vi "PathSearch.vi"(4 "Look-Ahead Time (s)":dbl=0.25, 6 "Search Window (s)":dbl=2.0, 8 "Robot Y (in)":dbl, 9 "Robot X (in)":dbl, 11 "Path":dbl[][](array[numeric])) -> (0 "Angle Goal (deg)":dbl, 1 "Velocity Goal (in/s)":dbl, 2 "Angle To Goal (deg)":dbl, 3 "Distance to Goal (in)":dbl, 5 "Distance from End (in)":dbl, 7 "Distance from Start (in)":dbl)   [LabVIEW 2018]
panel:
  out "Look-Ahead Point":i32
  out "Closest Point":i32
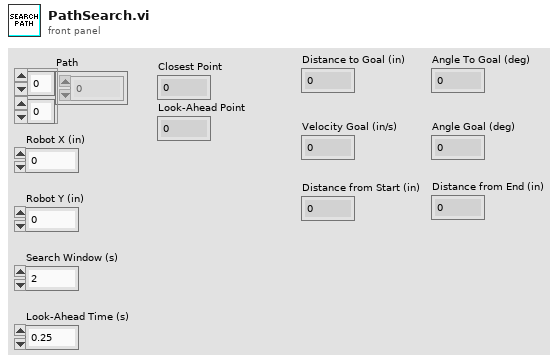
[diagram p1: front panel]
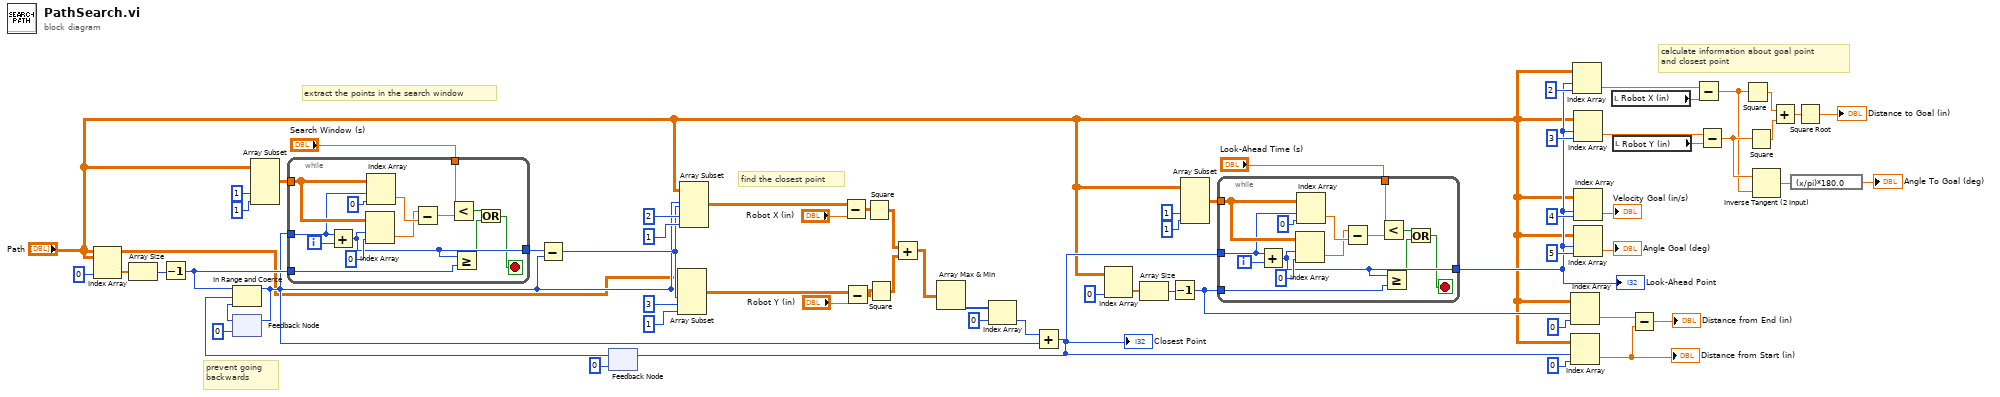
[diagram p0: block diagram]
diagram:
  # "calculate information about goal point\nand closest point"
  # "prevent going \nbackwards"
  # "find the closest point"
  # "extract the points in the search window"
  n1 = Index Array(array="Path", index (col)=0 ("disabled index (col)")) -> (element=w27:dbl[])  [unwired: 1 in]
  n2 = Array Size(array=w27) -> (size(s)=w28:i32)
  n3 = Decrement(x=w28) -> (x-1=w24:i32)
  n4 = feedback #1(0) -> (w25:i32)
  n5 = Array Subset(array="Path", index (col)=1 ("index"), length (col)=1 ("length")) -> (w48:dbl[][])  [unwired: 2 in]
  n6 = feedback #2(0) -> (w22:i32)
  n7 = In Range and Coerce(upper limit=w24, x=w22, lower limit=w25) -> (coerced(x)=w23:i32)  [unwired: 1 out]
  n8 = feedback-in #1(w23) -> ()
  n9 = while {
    tunnel: w23 -> [w76]
    tunnel: w48 -> [w77]
    tunnel: "Search Window (s)" -> [w71]
    tunnel: [w70] -> w46
    tunnel: w24 -> [w66]
    i -> [w79]
    stop <- w68 stop-if-true
    # "Search window"
    n10 = Add(x=w76, y=w79) -> (x+y=w70:i32)
    n11 = Index Array(array=w77, index (row)=w70, index (col)=0 ("disabled index (col)")) -> (element=w73:dbl)
    n12 = Index Array(array=w77, index (row)=w76, index (col)=0 ("disabled index (col)")) -> (element=w74:dbl)
    n13 = Subtract(x=w73, y=w74) -> (x-y=w72:dbl)
    n14 = Less?(x=w71, y=w72) -> (x < y?=w69:bool)
    n15 = Greater Or Equal?(x=w70, y=w66) -> (x >= y?=w67:bool)
    n16 = Or(x=w69, y=w67) -> (x .or. y?=w68:bool)
  }
  n17 = Subtract(x=w46, y=w23) -> (x-y=w45:i32)
  n18 = Array Subset(array="Path", index (row)=w23, length (row)=w45, index (col)=3 ("index"), length (col)=1 ("length")) -> (w57:dbl[][])
  n19 = Array Subset(array="Path", index (row)=w23, length (row)=w45, index (col)=2 ("index"), length (col)=1 ("length")) -> (w63:dbl[][])
  n20 = Subtract(x=w63, y="Robot X (in)") -> (x-y=w62:dbl[][])
  n21 = Subtract(x=w57, y="Robot Y (in)") -> (x-y=w58:dbl[][])
  n22 = Square(x=w62) -> (x^2=w55:dbl[][])
  n23 = Square(x=w58) -> (x^2=w54:dbl[][])
  n24 = Add(x=w55, y=w54) -> (x+y=w53:dbl[][])
  n25 = Array Max & Min(array=w53) -> (min index (indices)=w52:i32[])  [unwired: 3 out]
  n26 = Index Array(array=w52, index=0) -> (element=w44:i32)
  n27 = Add(x=w44, y=w23) -> (x+y=w9:i32)
  "Closest Point" <- w9
  n28 = feedback-in #2(w9) -> ()
  n29 = Index Array(array="Path", index (col)=0 ("disabled index (col)")) -> (element=w16:dbl[])  [unwired: 1 in]
  n30 = Array Size(array=w16) -> (size(s)=w8:i32)
  n31 = Decrement(x=w8) -> (x-1=w6:i32)
  n32 = Array Subset(array="Path", index (col)=1 ("index"), length (col)=1 ("length")) -> (w18:dbl[][])  [unwired: 2 in]
  n33 = while {
    tunnel: w9 -> [w90]
    tunnel: w18 -> [w91]
    tunnel: "Look-Ahead Time (s)" -> [w85]
    tunnel: [w84] -> w10
    tunnel: w6 -> [w80]
    i -> [w93]
    stop <- w82 stop-if-true
    # "Search window"
    n34 = Add(x=w90, y=w93) -> (x+y=w84:i32)
    n35 = Index Array(array=w91, index (row)=w84, index (col)=0 ("disabled index (col)")) -> (element=w87:dbl)
    n36 = Index Array(array=w91, index (row)=w90, index (col)=0 ("disabled index (col)")) -> (element=w88:dbl)
    n37 = Subtract(x=w87, y=w88) -> (x-y=w86:dbl)
    n38 = Less?(x=w85, y=w86) -> (x < y?=w83:bool)
    n39 = Greater Or Equal?(x=w84, y=w80) -> (x >= y?=w81:bool)
    n40 = Or(x=w83, y=w81) -> (x .or. y?=w82:bool)
  }
  "Look-Ahead Point" <- w10
  n41 = Index Array(array="Path", index (row)=w6, index (col)=0 ("disabled index (row)")) -> (element=w4:dbl)
  n42 = Index Array(array="Path", index (row)=w9, index (col)=0 ("disabled index (col)")) -> (element=w2:dbl)
  "Distance from Start (in)" <- w2
  n43 = Index Array(array="Path", index (row)=w10, index (col)=2 ("disabled index (col)")) -> (element=w41:dbl)
  n44 = Index Array(array="Path", index (row)=w10, index (col)=3 ("disabled index (col)")) -> (element=w39:dbl)
  n45 = Index Array(array="Path", index (row)=w10, index (col)=4 ("disabled index (col)")) -> (element=→"Velocity Goal (in/s)":dbl)
  n46 = Index Array(array="Path", index (row)=w10, index (col)=5 ("disabled index (col)")) -> (element=→"Angle Goal (deg)":dbl)
  n47 = local read "Robot X (in)"() -> (w40:dbl)
  n48 = local read "Robot Y (in)"() -> (w38:dbl)
  n49 = Subtract(x=w4, y=w2) -> (x-y=→"Distance from End (in)":dbl)
  n50 = Subtract(x=w41, y=w40) -> (x-y=w32:dbl)
  n51 = Subtract(x=w39, y=w38) -> (x-y=w33:dbl)
  n52 = Square(x=w32) -> (x^2=w36:dbl)
  n53 = Square(x=w33) -> (x^2=w37:dbl)
  n54 = Inverse Tangent (2 Input)(1:w32, 2:w33) -> (0:w31:dbl)
  n55 = Add(x=w36, y=w37) -> (x+y=w35:dbl)
  n56 = expression code="(x/pi)*180.0"(w31) -> (→"Angle To Goal (deg)":dbl)
  n57 = Square Root(x=w35) -> (sqrt(x)=→"Distance to Goal (in)":dbl)
